vi "App Queue Instances.vi"   [LabVIEW 2019]
uses:
  Message Queue.lvlib
  Status/Status.lvlib
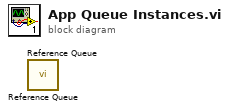
[diagram p0: block diagram]
diagram:
  n1 = call "Reference Queue.vi"() -> ()  [unwired: 11 in, 1 out]
  n2 = call "Reference Queue.vi"() -> ()  [unwired: 11 in, 1 out]
